vi "getProcessViPath.vi"(7 "Enum Screen":T1, 8 "error in (no error)":errorcluster) -> (0 "error out":errorcluster, 3 "Path":path)   [LabVIEW 2011]
uses:
  EnumProcess.ctl
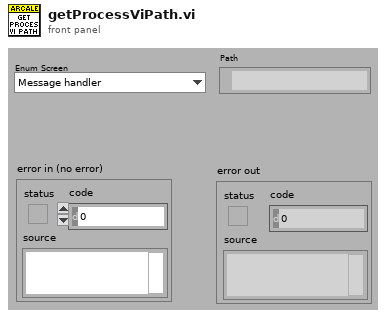
[diagram p1: front panel]
types:
  T1 = typedef "EnumProcess.ctl" = enum16{"Message handler", "Template"}
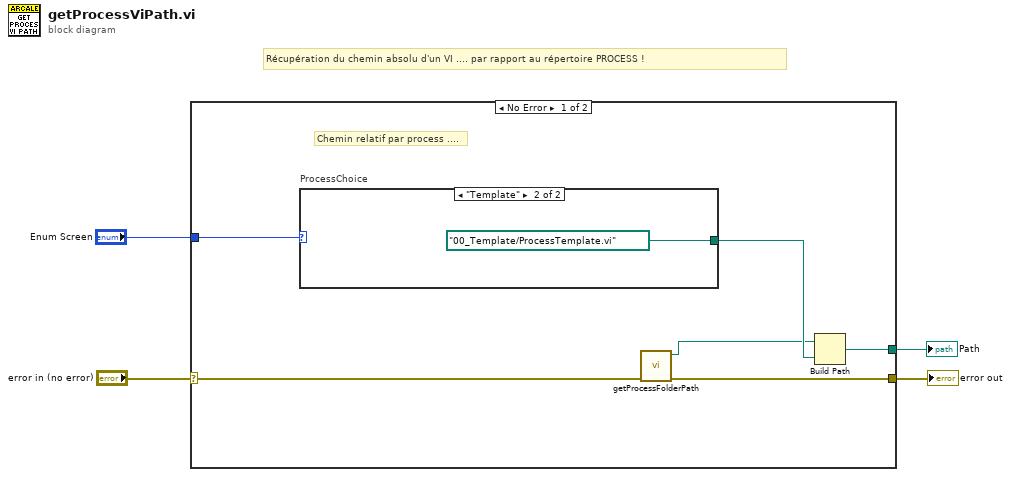
[diagram p0: block diagram]
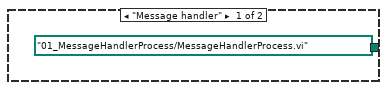
[diagram p2: hidden frame]
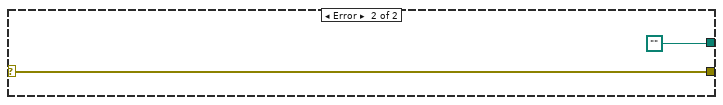
[diagram p3: hidden frame]
diagram:
  # "Récupération du chemin absolu d'un VI .... par rapport au répertoire PROCESS !"
  n1 = case shown="No Error" "error in (no error)" {
    selector: "error in (no error)" -> [w7 w14]
    tunnel: [w6 w14] -> w4
    tunnel: "Enum Screen" -> [w10 _]
    tunnel: [w9 path ""] -> w1
    frame No Error {
      # "Chemin relatif par process ...."
      n2 = case "ProcessChoice" shown="\"Template\"" w10 {
        tunnel: [path "01_MessageHandlerProcess/MessageHandlerProcess.vi" ("path") path "00_Template/ProcessTemplate.vi" ("path")] -> w8
        frame "Message handler" {
        }
        frame "Template" {
        }
      }
      n3 = call "getProcessFolderPath.vi"("error in (no error)"=w7) -> ("error out"=w6:errorcluster, "Process Folder"=w5:path)  [unwired: 9 in]
      n4 = Build Path(base path=w5, name or relative path=w8) -> (appended path=w9:path)
    }
    frame Error {
    }
  }
  "error out" <- w4
  "Path" <- w1
